vi "Zero Steer Jaguars.vi"() -> ()   [LabVIEW 2012]
uses:
  Controls/Zero Steer Jags Shifter.ctl
  <vilib>/Rock Robotics/SystemInterfaces/Utilities/FPGA_UtilitiesLED Source.ctl
  <vilib>/Rock Robotics/SystemInterfaces/Utilities/FPGA_UtilitiesLED State.ctl
  Globals/Potentiometers.vi
  <vilib>/Rock Robotics/WPI/Joystick/WPI_JoystickGetSetRefNum.vi
  Globals/Are We Calibrating Steering.vi
  Globals/Jaguar Commands.vi
  Globals/Motor Errors.vi
  Globals/Max Steer Voltage.vi
  <vilib>/Utility/file.llb/Write To Spreadsheet File (DBL).vi
  Globals/Pot Home Values.vi
panel:
  in  "Max Voltage":dbl
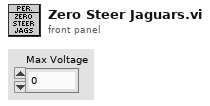
[diagram p1: front panel]
types:
  T1 = typedef "Zero Steer Jags Shifter.ctl" = enum16{"Wait for Button", "Move to Halfway", "Wait for Record"}
  T2 = typedef "WPI_AnalogChannelDevRef.ctl" = cluster{"DevStatus":errorcluster, "Analog Module":T3, "Analog Channel":T4}
  T3 = typedef "FPGA_TypedefAnalogModule.ctl" = enum16{"Analog Module 1", "Analog Module 2"}
  T4 = typedef "FPGA_AIChannel.ctl" = enum8{"AI 1", "AI 2", "AI 3", "AI 4", "AI 5", "AI 6", "AI 7", "AI 8", "Invalid"}
  T5 = cluster{"Front Left":T2, "Front Right":T2, "Rear Left":T2, "Rear Right":T2, "Actuator":T2}
  T6 = typedef "WPI_JoystickDevRef.ctl" = cluster{"Device":T7}
  T7 = typedef "WPI_JoystickDeviceEnum.ctl" = enum16{"USB 1", "USB 2", "USB 3", "USB 4", "Kinect 1", "Kinect 2"}
  T8 = typedef "FPGA_UtilitiesLED State.ctl" = enum16{"Off", "On", "Toggle"}
  T9 = typedef "FPGA_UtilitiesLED Source.ctl" = enum16{"User LED", "FPGA LED"}
  T10 = typedef "WPI_JoystickButtonState.ctl" = cluster{"Button 1":bool, "Button 2":bool, "Button 3":bool, "Button 4":bool, "Button 5":bool, "Button 6":bool, "Button 7":bool, "Button 8":bool, "Button 9":bool, "Button 10":bool, "Button 11":bool, "Button 12":bool}
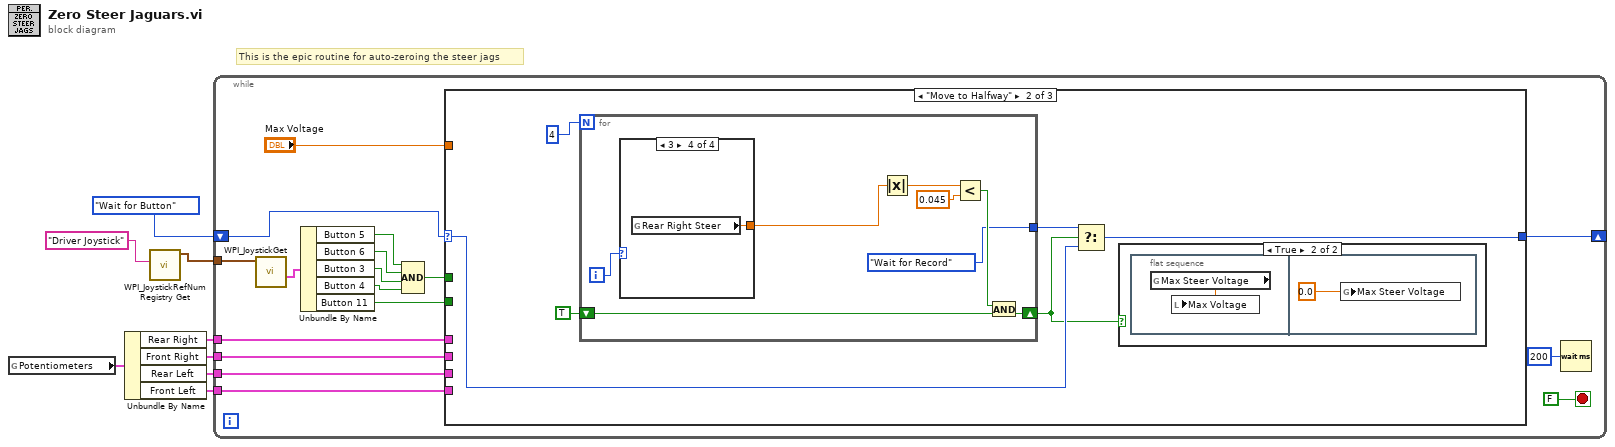
[diagram p0: block diagram]
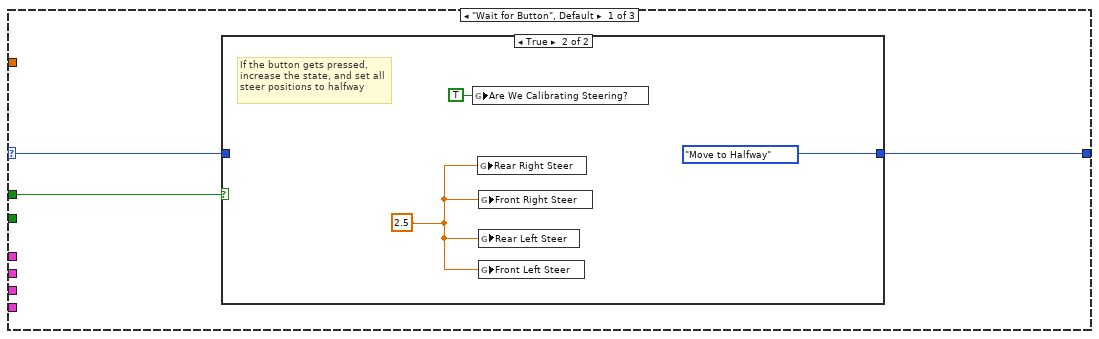
[diagram p2: hidden frame]
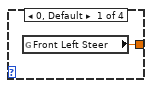
[diagram p5: hidden frame]
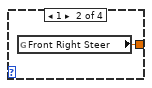
[diagram p6: hidden frame]
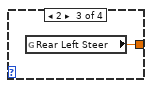
[diagram p7: hidden frame]
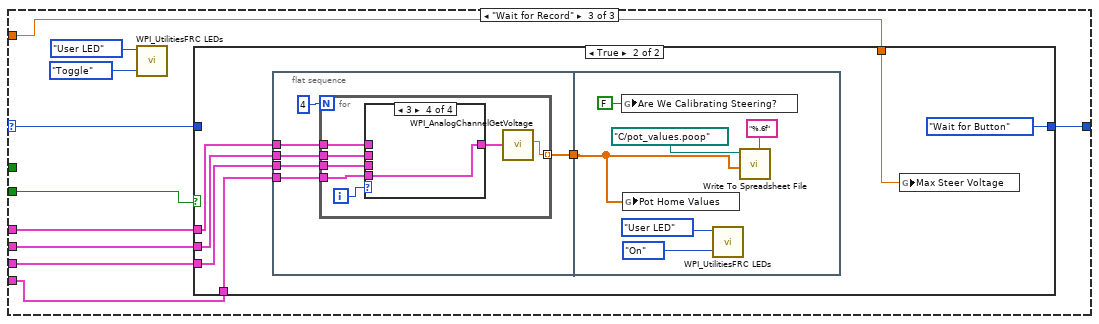
[diagram p8: hidden frame]
diagram:
  # "This is the epic routine for auto-zeroing the steer jags"
  n1 = global read "Potentiometers.vi" "Potentiometers"() -> (w5:T5)
  n2 = Unbundle By Name(w5) -> ("Rear Right"=w4:T2, "Front Right"=w3:T2, "Rear Left"=w2:T2, "Front Left"=w1:T2)
  n3 = call <vilib>:"WPI_JoystickRefNum Registry Get.vi"("refnum name"="Driver Joystick") -> ("JoystickDevRef"=w8:T6)  [unwired: 1 in, 9 out]
  n4 = while {
    tunnel: w8 -> [w19]
    shift-right: [w23] -> _
    shift-left: Zero_Steer_Jags_Shifter."Wait for Button" ("States") -> [w24]
    tunnel: w4 -> [w12]
    tunnel: w3 -> [w11]
    tunnel: w2 -> [w10]
    tunnel: w1 -> [w9]
    stop <- FALSE stop-if-true
    n5 = call <vilib>:"WPI_JoystickGet.vi"("JoystickDevRef"=w19) -> ("Buttons"=w21:T10)  [unwired: 4 in, 2 out]
    n6 = Unbundle By Name(w21) -> ("Button 5"=w17:bool, "Button 6"=w16:bool, "Button 3"=w20:bool, "Button 4"=w15:bool, "Button 11"=w14:bool)
    n7 = Compound Arithmetic op=AND(w17, w16, w20, w15) -> (w18:bool)
    n8 = case shown="\"Move to Halfway\"" w24 {
      selector: w24 -> [w28 w35 w60]
      tunnel: [w27 w36 w59] -> w23
      tunnel: w18 -> [w26 _ _]
      tunnel: w14 -> [_ _ w58]
      tunnel: w12 -> [_ _ w57]
      tunnel: w11 -> [_ _ w56]
      tunnel: w10 -> [_ _ w55]
      tunnel: w9 -> [_ _ w54]
      tunnel: "Max Voltage" -> [_ _ w53]
      frame "Wait for Button", Default {
        n9 = case shown="True" w26 {
          tunnel: w28 -> [w29 _]
          tunnel: [w29 Zero_Steer_Jags_Shifter."Move to Halfway" ("States")] -> w27
          frame False {
          }
          frame True {
            w30 = 2.5 ("Front Right Steer")
            # "If the button gets pressed, \nincrease the state, and set all\nsteer positions to halfway"
            n10 = global write "Are We Calibrating Steering.vi" "Are We Calibrating Steering?"(TRUE ("Are We Calibrating Steering?")) -> ()
            n11 = global write "Jaguar Commands.vi" "Rear Right Steer"(w30) -> ()
            n12 = global write "Jaguar Commands.vi" "Front Right Steer"(w30) -> ()
            n13 = global write "Jaguar Commands.vi" "Rear Left Steer"(w30) -> ()
            n14 = global write "Jaguar Commands.vi" "Front Left Steer"(w30) -> ()
          }
        }
      }
      frame "Move to Halfway" {
        n15 = for {
          N: 4 -> [_]
          shift-right: [w46] -> w33
          shift-left: TRUE -> [w45]
          tunnel: [Zero_Steer_Jags_Shifter."Wait for Record" ("States")] -> w34
          i -> [w48]
          n16 = case shown="3" w48 {
            tunnel: [w49 w50 w51 w52] -> w41
            frame 0, Default {
              n17 = global read "Motor Errors.vi" "Front Left Steer"() -> (w49:dbl)
            }
            frame 1 {
              n18 = global read "Motor Errors.vi" "Front Right Steer"() -> (w50:dbl)
            }
            frame 2 {
              n19 = global read "Motor Errors.vi" "Rear Left Steer"() -> (w51:dbl)
            }
            frame 3 {
              n20 = global read "Motor Errors.vi" "Rear Right Steer"() -> (w52:dbl)
            }
          }
          n21 = Absolute Value(x=w41) -> (abs(x)=w42:dbl)
          n22 = Less?(x=w42, y=0.045) -> (x < y?=w44:bool)
          n23 = And(x=w44, y=w45) -> (x .and. y?=w46:bool)
        }
        n24 = Select(t=w34, s=w33, f=w35) -> (s? t:f=w36:T1)
        n25 = case shown="True" w33 {
          frame False {
          }
          frame True {
            n26 = flat-sequence {
              frame #0 {
                n27 = global read "Max Steer Voltage.vi" "Max Steer Voltage"() -> (w39:dbl)
                n28 = local write "Max Voltage"(w39) -> ()
              }
              frame #1 {
                n29 = global write "Max Steer Voltage.vi" "Max Steer Voltage"(0.0 ("Max Steer Voltage")) -> ()
              }
            }
          }
        }
      }
      frame "Wait for Record" {
        n30 = call <vilib>:"WPI_UtilitiesFRC LEDs.vi"("State"=FPGA_UtilitiesLED_State."Toggle", "LED Type"=FPGA_UtilitiesLED_Source."User LED") -> ()  [unwired: 8 in, 2 out]
        n31 = case shown="True" w58 {
          tunnel: w60 -> [w63 _]
          tunnel: [w63 Zero_Steer_Jags_Shifter."Wait for Button" ("States")] -> w59
          tunnel: w57 -> [_ w69]
          tunnel: w56 -> [_ w68]
          tunnel: w55 -> [_ w67]
          tunnel: w54 -> [_ w66]
          tunnel: w53 -> [_ w64]
          frame False {
          }
          frame True {
            n32 = flat-sequence {
              tunnel: w69 -> [w75]
              tunnel: w68 -> [w74]
              tunnel: w67 -> [w73]
              tunnel: w66 -> [w72]
              tunnel: [w71] -> w65
              tunnel: w65 -> [w88]
              frame #0 {
                n33 = for {
                  N: 4 -> [_]
                  tunnel: w75 -> [w82]
                  tunnel: w74 -> [w81]
                  tunnel: w73 -> [w80]
                  tunnel: w72 -> [w79]
                  tunnel: [w77] -> w71 mode=indexing
                  i -> [w83]
                  n34 = case shown="3" w83 {
                    tunnel: w82 -> [w84 _ _ _]
                    tunnel: w81 -> [_ w85 _ _]
                    tunnel: w80 -> [_ _ w86 _]
                    tunnel: w79 -> [_ _ _ w87]
                    tunnel: [w84 w85 w86 w87] -> w78
                    frame 0, Default {
                    }
                    frame 1 {
                    }
                    frame 2 {
                    }
                    frame 3 {
                    }
                  }
                  n35 = call <vilib>:"WPI_AnalogChannelGetVoltage.vi"("AIDeviceRef"=w78) -> ("Voltage"=w77:dbl)  [unwired: 8 in, 2 out]
                }
              }
              frame #1 {
                n36 = global write "Are We Calibrating Steering.vi" "Are We Calibrating Steering?"(FALSE ("Are We Calibrating Steering?")) -> ()
                n37 = global write "Pot Home Values.vi" "Pot Home Values"(w88) -> ()
                n38 = call <vilib>:"WPI_UtilitiesFRC LEDs.vi"("State"=FPGA_UtilitiesLED_State."On", "LED Type"=FPGA_UtilitiesLED_Source."User LED") -> ()  [unwired: 8 in, 2 out]
                n39 = call-poly <vilib>:"Write To Spreadsheet File.vi"("format (%.3f)"="%.6f", "1D data"=w88, "file path (dialog if empty)"=path "C:/pot_values.poop") -> ()  [unwired: 5 in, 1 out]
              }
            }
            n40 = global write "Max Steer Voltage.vi" "Max Steer Voltage"(w64) -> ()
          }
        }
      }
    }
    n41 = Wait (ms)(milliseconds to wait=u32 200) -> ()  [unwired: 1 out]
  }
